vi "Init.vi"(8 "error in (no error)":errorcluster, 10 "Product_Ref":string, 11 "Board in":refnum<class "Board.lvclass">) -> (0 "error out":errorcluster, 3 "Board out":refnum<class "Board.lvclass">)   [LabVIEW 2025, in "SW License Manager.lvlib" / "Board.lvclass"]
uses:
  Board.lvclass
  <vilib>/Utility/error.llb/Error Cluster From Error Code.vi
  <vilib>/ErrorRing/Error Ring.xnode
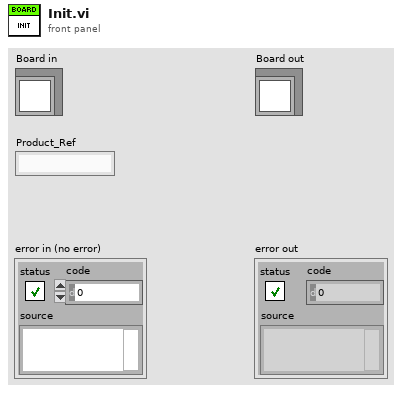
[diagram p1: front panel]
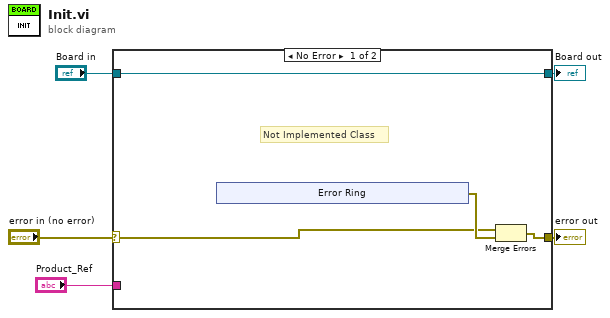
[diagram p0: block diagram]
diagram:
  n1 = case shown="No Error" "error in (no error)" {
    selector: "error in (no error)" -> [w6 w15]
    tunnel: [w7 w15] -> w3
    tunnel: [w9 w14] -> w2
    tunnel: "Board in" -> [w9 w14]
    tunnel: "Product_Ref" -> [_ _]
    frame No Error {
      # "Not Implemented Class"
      n2 = xnode "Error Ring"() -> ("error out"=w8:errorcluster)
      n3 = Merge Errors(w6, w8) -> (w7:errorcluster)
    }
    frame Error {
    }
  }
  "error out" <- w3
  "Board out" <- w2
